vi "c_ctre_phoenix6_platform_write_integer.vi"(0 "String":string, 1 "Numeric 2":i64, 2 "String 2":string, 3 "Numeric 3":dbl) -> (20 "Numeric":i32)   [LabVIEW 2023]
uses:
  <vilib>/Rock Robotics/WPI/ThirdParty/Phoenix-LabVIEW/Controls/DriverLib.ctl
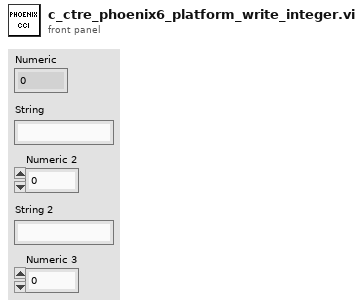
[diagram p1: front panel]
types:
  T1 = typedef "DriverLib.ctl" = path
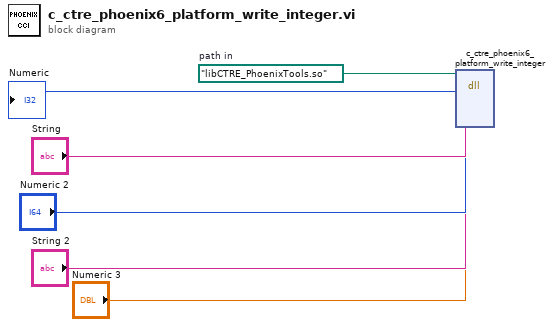
[diagram p0: block diagram]
diagram:
  w6 = T1 path "libCTRE_PhoenixTools.so"  # path in
  n1 = dll-call lib="?" fn="c_ctre_phoenix6_platform_write_integer"(path in=w6, "String", "Numeric 2", "String 2", "Numeric 3") -> (→"Numeric":i32)  [unwired: 6 in, 2 out]
